vi "Initialize_ErrorHandler.vi"(8 "error in (no error)":errorcluster) -> (0 "error out":errorcluster, 3 "ErrorHandler out":refnum<class "ErrorHandler.lvclass">)   [LabVIEW 2017, in "ErrorHandler.lvclass"]
doc: "Developed by Kevin Thompson\nkevin@thompsonengineering.net\n\nCopyright 2018\nThompson Engineering, LLC"
uses:
  ErrorHandler.lvclass
  TypeDef/ErrorRemote EventData.ctl
  TypeDef/ObjData--cluster.ctl
  TypeDef/TD GetSet ActionSelect--enum.ctl
  ErrorHandler.lvclass/ErrorHandler.ctl
  Accessors/Set DialogDisabled.vi
  Accessors/Set TerminateEnabled.vi
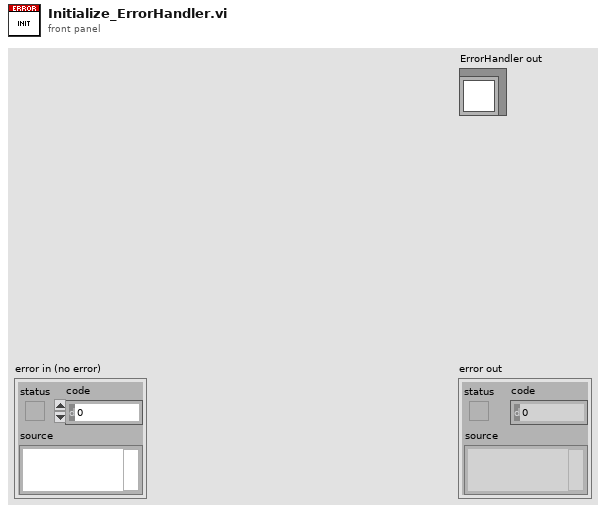
[diagram p1: front panel]
types:
  T1 = typedef "ErrorHandler.lvclass/TD GetSet ActionSelect--enum.ctl" = enum16{"Init", "Get", "Set"}
  T2 = typedef "ErrorHandler.lvclass/ObjData--cluster.ctl" = cluster{"AppName":string, "ErrorLogBasePath":path, "ErrorDialogPopUp Disabled":bool, "TerminateAppOnError Enabled":bool}
  T3 = typedef "ErrorHandler.lvclass/ErrorRemote EventData.ctl" = cluster{"Timestamp":timestamp, "ErrorCluster":errorcluster, "message":string, "Shutdown?":bool, "DialogDisabled?":bool, "TerminateOnError?":bool}
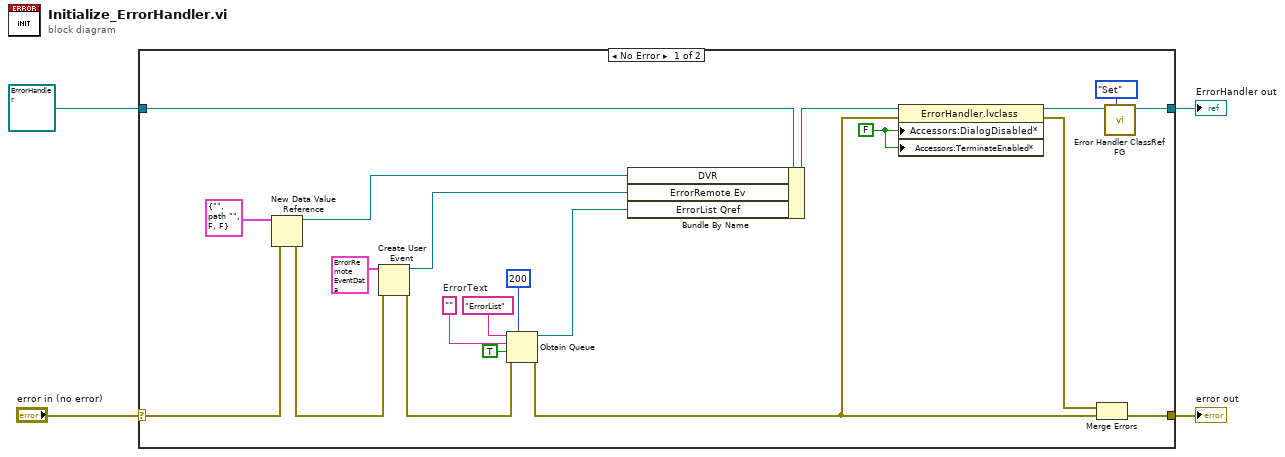
[diagram p0: block diagram]
diagram:
  n1 = case shown="No Error" "error in (no error)" {
    selector: "error in (no error)" -> [w17 w27]
    tunnel: [w10 w27] -> w3
    tunnel: [w5 w26] -> w1
    tunnel: refnum<class "ErrorHandler.lvclass"> refnum ("ErrorHandler in") -> [w25 w26]
    frame No Error {
      w11 = FALSE ("DialogEnabled*")
      w22 = ""  # ErrorText
      n2 = New Data Value Reference(data value=T2 {"AppName"="", "ErrorLogBasePath"=path "", "ErrorDialogPopUp Disabled"=FALSE, "TerminateAppOnError Enabled"=FALSE} ("ObjData"), error in=w17) -> (data value reference=w15:refnum<data-value>, error out=w16:errorcluster)
      n3 = Create User Event(user event datatype=T3 {"Timestamp"=timestamp(0 s since 1904-01-01), "ErrorCluster"={"status"=FALSE, "code"=0, "source"=""}, "message"="", "Shutdown?"=FALSE, "DialogDisabled?"=FALSE, "TerminateOnError?"=FALSE} ("ErrorRemote"), error in=w16) -> (user event=w23:refnum<user-event>, error out=w19:errorcluster)
      n4 = Obtain Queue(max queue size (-1, unlimited)=200, name (unnamed)="ErrorList", element data type=w22, create if not found? (T)=TRUE, error in (no error)=w19) -> (queue out=w18:refnum<queue>, error out=w8:errorcluster)  [unwired: 1 out]
      n5 = Bundle By Name(cluster=w25, "DVR"=w15, "ErrorRemote Ev"=w23, "ErrorList Qref"=w18) -> (w12:refnum<class "ErrorHandler.lvclass">)
      n6 = property class="ErrorHandler.lvclass"(reference=w12, error in=w8, "Accessors:DialogDisabled*"=w11, "Accessors:TerminateEnabled*"=w11) -> (reference out=w6:refnum<class "ErrorHandler.lvclass">, error out=w9:errorcluster)
      n7 = Merge Errors(w9, w8) -> (w10:errorcluster)
      n8 = call "Error Handler ClassRef FG.vi"("action (Get)"=TD_GetSet_ActionSelect--enum."Set", "ErrorHandler in"=w6) -> ("ErrorHandler out"=w5:refnum<class "ErrorHandler.lvclass">)  [unwired: 8 in, 1 out]
    }
    frame Error {
    }
  }
  "error out" <- w3
  "ErrorHandler out" <- w1
